vi "Auto Sequencing.vi"(11 "DaqControl in":T1) -> (3 "DaqControl out":T1)   [LabVIEW 2020, in "VolatusDaq.lvlib" / "DaqControl.lvclass"]
uses:
  DaqControl.lvclass
  DaqControl.lvclass/DaqControl.ctl
  Value Update.ctl
  Sequence Action.ctl
  VolatusDaq.lvlib
  Loop Data.ctl
  Seq Cmd Type.ctl
  Seq Action Type.ctl
  Seq Cmd.ctl
  Signal Type.ctl
  Volatus/Event API/EventAPI.lvclass
  Volatus/DataHandlerAPI/DataHandlerAPI.lvclass
  Sequence.ctl
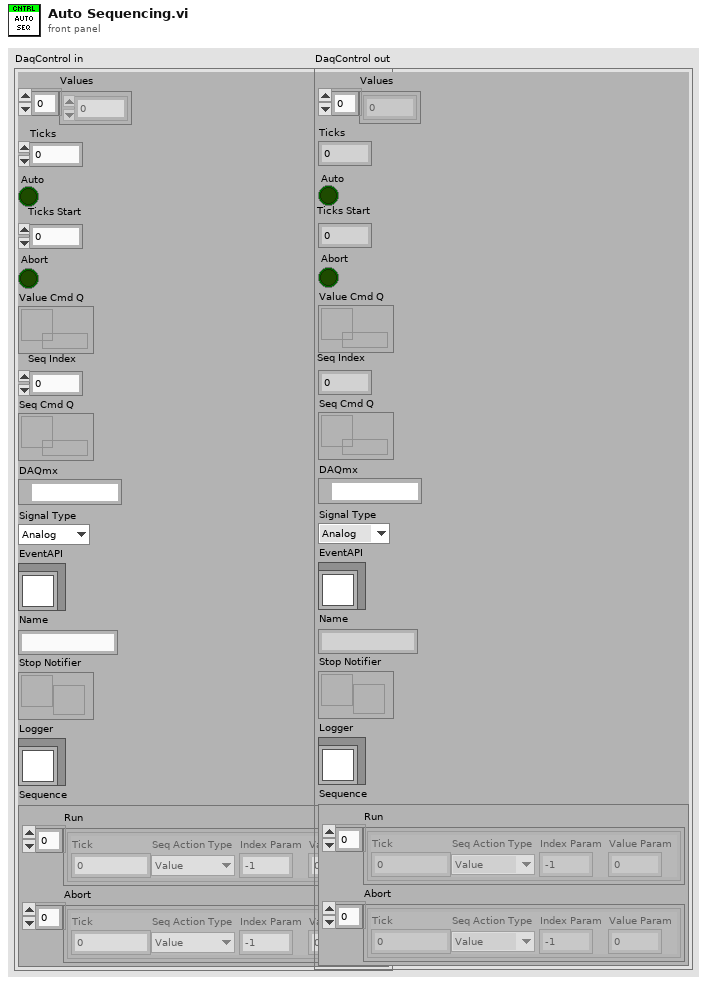
[diagram p1: front panel]
types:
  T1 = typedef "VolatusDaq.lvlib/DaqControl.lvclass/Loop Data.ctl" = cluster{"Values":dbl[], "Ticks":u32, "Auto":bool, "Ticks Start":u32, "Abort":bool, "Value Cmd Q":refnum<queue>, "Seq Index":i32, "Seq Cmd Q":refnum<queue>, "DAQmx":refnum<k21>, "Signal Type":T2, "EventAPI":refnum<class "EventAPI.lvclass">, "Name":string, "Stop Notifier":refnum<notifier>, "Logger":refnum<class "DataHandlerAPI.lvclass">, "Sequence":T3}
  T2 = typedef "VolatusDaq.lvlib/Signal Type.ctl" = enum16{"Analog", "Digital"}
  T3 = typedef "VolatusDaq.lvlib/Sequence.ctl" = cluster{"Run":T4[], "Abort":T4[]}
  T4 = typedef "VolatusDaq.lvlib/Sequence Action.ctl" = cluster{"Tick":u32, "Seq Action Type":T5, "Index Param":i32, "Value Param":dbl}
  T5 = typedef "VolatusDaq.lvlib/Seq Action Type.ctl" = enum16{"Value", "Stop"}
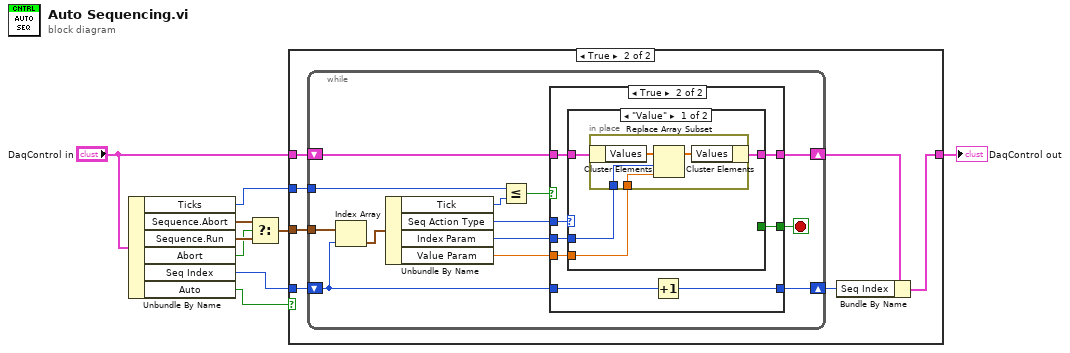
[diagram p0: block diagram]
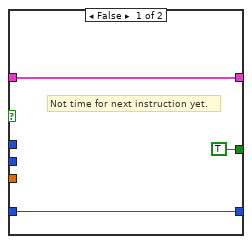
[diagram p3: hidden frame]
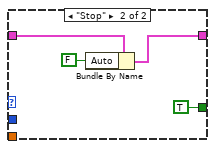
[diagram p4: hidden frame]
diagram:
  n1 = Unbundle By Name("DaqControl in") -> ("Ticks"=w1:u32, "Sequence.Abort"=w5:T4[], "Sequence.Run"=w4:T4[], "Abort"=w3:bool, "Seq Index"=w7:i32, "Auto"=w9:bool)
  n2 = Select(t=w5, s=w3, f=w4) -> (s? t:f=w2:T4[])
  n3 = case shown="True" w9 {
    tunnel: "DaqControl in" -> [w10 w17]
    tunnel: [w10 w11] -> w8
    tunnel: w7 -> [_ w16]
    tunnel: w2 -> [_ w15]
    tunnel: w1 -> [_ w14]
    frame False {
    }
    frame True {
      n4 = while {
        shift-right: [w29] -> w13
        shift-left: w17 -> [w30]
        shift-right: [w19] -> w12
        shift-left: w16 -> [w27]
        tunnel: w15 -> [w28]
        tunnel: w14 -> [w25]
        stop <- w18 stop-if-true
        n5 = Index Array(array=w28, index=w27) -> (element=w26:T4)
        n6 = Unbundle By Name(w26) -> ("Tick"=w24:u32, "Seq Action Type"=w23:T5, "Index Param"=w22:i32, "Value Param"=w21:dbl)
        n7 = Less Or Equal?(x=w25, y=w24) -> (x <= y?=w20:bool)
        n8 = case shown="True" w20 {
          tunnel: w30 -> [w33 w41]
          tunnel: [w33 w40] -> w29
          tunnel: w27 -> [w32 w36]
          tunnel: w23 -> [_ w39]
          tunnel: w22 -> [_ w38]
          tunnel: w21 -> [_ w37]
          tunnel: [w32 w35] -> w19
          tunnel: [TRUE w34] -> w18
          frame False {
            # "Not time for next instruction yet."
          }
          frame True {
            n9 = case shown="\"Value\"" w39 {
              tunnel: w41 -> [w45 w53]
              tunnel: [w44 w51] -> w40
              tunnel: w38 -> [w43 _]
              tunnel: w37 -> [w42 _]
              tunnel: [_ TRUE] -> w34
              frame "Value" {
                n10 = in-place {
                  in-place-border: w43 -> [w47]
                  in-place-border: w42 -> [w46]
                  n11 = in-place-cluster #1(w45) -> ("Values"=w49:dbl[])
                  n12 = Replace Array Subset(array=w49, new element=w46, index=w47) -> (w48:dbl[])
                  n13 = in-place-cluster #1("Values"=w48) -> (w44:T1)
                }
              }
              frame "Stop" {
                n14 = Bundle By Name(cluster=w53, "Auto"=FALSE) -> (w51:T1)
              }
            }
            n15 = Increment(x=w36) -> (x+1=w35:i32)
          }
        }
      }
      n16 = Bundle By Name(cluster=w13, "Seq Index"=w12) -> (w11:T1)
    }
  }
  "DaqControl out" <- w8
